vi "RT_Lissajou_fit_Oct.vi"() -> ()   [LabVIEW 2019]
uses:
  <vilib>/Platform/TimedLoop/XDataNode/timing_clust.ctl
  <vilib>/Platform/TimedLoop/XDataNode/nitl_modes.ctl
  <vilib>/Platform/TimedLoop/XDataNode/wakeup.ctl
  <vilib>/FPGAPlugInAG/myRIO-1900/niLvFpga_Open_myRIO-1900.vi
  <vilib>/rvi/interface/common/dynamic/niFpgaDynamicAddResources.vi
  <vilib>/Utility/error.llb/Error Cluster From Error Code.vi
  <vilib>/rvi/errors/niLvFpgaAdjustHostInterfaceError.vi
  <vilib>/gmath/NumericalOptimization/Nonlinear Curve Fit LM.vi
  <vilib>/platform/TimedLoop/XDataNode/XDataNode.xnode
  <vilib>/rvi/interface/nirviOpenFPGA/nirviOpenFPGA.xnode
  FPGA Bitfiles/studentchallenge_FPGATarget_FPGA1RADC1WDAC2A_GeAN6BgpSew.lvbitx
  <vilib>/rvi/interface/nirviReadWriteControl/nirviReadWriteControl.xnode
  <vilib>/Platform/TimedLoop/XDataNode/XDNodeRunTimeDep.lvlib
  <vilib>/gmath/NI_Gmath.lvlib
  <vilib>/Analysis/NI_AALBase.lvlib
  <vilib>/rvi/interface/Simulation/niFpgaSimulationCallBeginRW.vi
  NiFpgaLv.dll
panel:
  out "Fit":cluster{"X":dbl[], "Y":dbl[]}[](graph)
  out "Fit parameters":dbl[](array[numeric])=[0.5568165492992482, 1.080914000787513, 2.5775367916302736, 1.4146358342436716, -0.5221777499831268]
  out "?":dbl(graph)=3.104248046875
  out "Finished Late? [i-1]":bool
  out "?":dbl(graph)=1.22314453125
  in  "stop":bool
  out "Lissajou":cluster{"X":dbl[], "Y":dbl[]}[](graph)
  in  "Loop time (us)":i64=2000
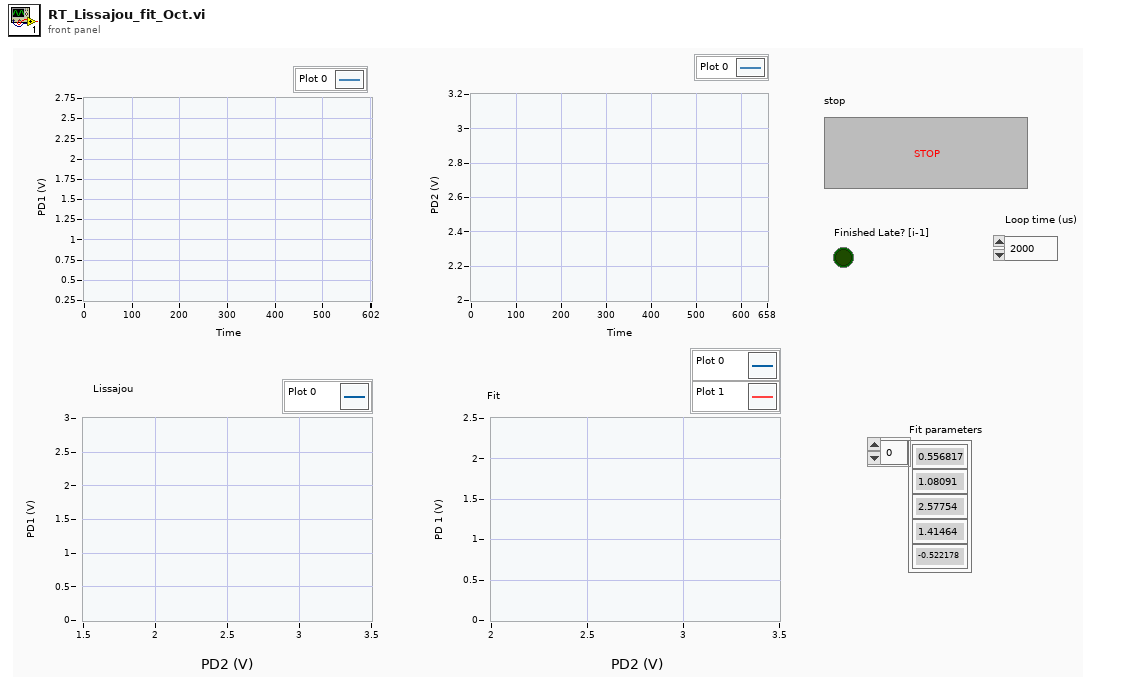
[diagram p1: front panel]
types:
  T1 = typedef "XDNodeRunTimeDep.lvlib/timing_clust.ctl" = cluster{"Expected End [f-1]":u64, "Actual End [f-1]":u64, "Finished Late? [f-1]":bool, "Expected End [i-1]":u64, "Actual End [i-1]":u64, "Finished Late? [i-1]":bool, "Expected Start [i]":u64, "Actual Start [i]":u64, "Expected Start [f]":u64, "Actual Start [f]":u64, "Source Name":string, "Structure Name":string, "Period":i64, "Deadline":i64, "Offset":i64, "Start":i64, "Priority":i32, "Timeout":i32, "Mode":T2, "Wakeup Reason":T3, "Error":errorcluster, "Source Type":string, "Secondary Source Type":string, "Global End Time":u64, "Global Start Time":u64, "Frame Duration":u64, "Iteration Duration":u64, "Assigned CPU":i32, "I/O Scan Engine Mode":u32}
  T2 = typedef "XDNodeRunTimeDep.lvlib/nitl_modes.ctl" = enum32{"No Change", "Process missed periods, maintain original phase", "Discard missed periods, maintain original phase", "Process missed periods, ignore original phase", "Discard missed periods, ignore original phase"}
  T3 = typedef "XDNodeRunTimeDep.lvlib/wakeup.ctl" = enum32{"Normal", "Aborted", "Asynchronous wakeup", "Timing source error", "Timed loop error", "Timeout"}
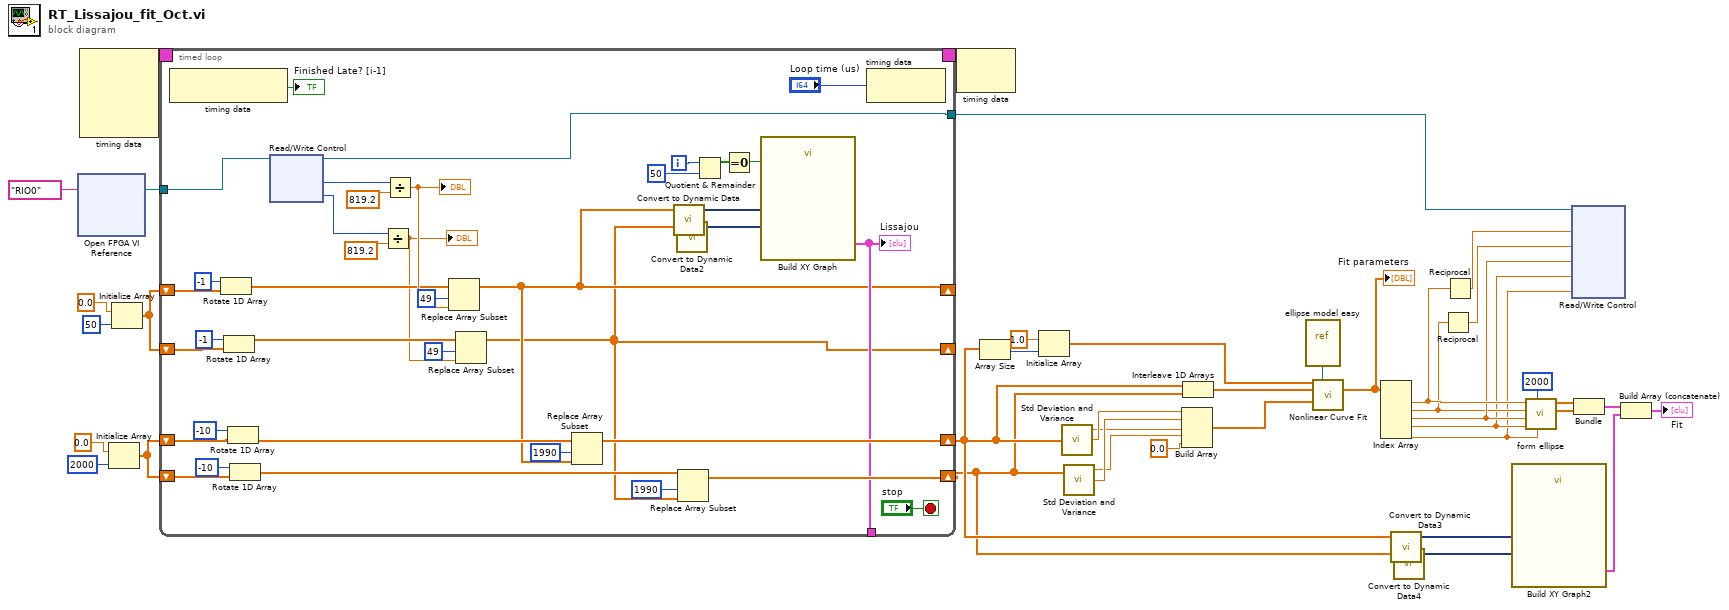
[diagram p0: block diagram]
diagram:
  n1 = xnode "Open FPGA VI Reference"("resource name"=tag "RIO0") -> ("FPGA VI Reference Out"=w37:refnum<k20>)  [unwired: 1 in, 1 out]
  n2 = node-c288() -> (w40:T1)  [unwired: 4 in]
  n3 = Initialize Array(0.0 ("element"), 2000 ("dimension size")) -> (w16:dbl[])
  n4 = Initialize Array(0.0 ("element"), 50 ("dimension size")) -> (w17:dbl[])
  n5 = timed-loop {
    timing: w40 -> [_]
    timing-out: [_] -> w39
    tunnel: w37 -> [w72]
    shift-right: [w43] -> _
    shift-left: w17 -> [w50]
    shift-right: [w44] -> _
    shift-left: w17 -> [w51]
    shift-right: [w49] -> w11
    shift-left: w16 -> [w48]
    shift-right: [w47] -> w12
    shift-left: w16 -> [w46]
    tunnel: [w45] -> _
    tunnel: [w41] -> w1
    i -> [w69]
    stop <- "stop" stop-if-true
    n6 = node-c288() -> (→"Finished Late? [i-1]":bool)  [unwired: 1 in]
    n7 = Rotate 1D Array(1:w51, 2:-1 ("n")) -> (0:w54:dbl[])
    n8 = Rotate 1D Array(1:w50, 2:-1 ("n")) -> (0:w53:dbl[])
    n9 = Rotate 1D Array(1:w46, 2:-10 ("n")) -> (0:w58:dbl[])
    n10 = Rotate 1D Array(1:w48, 2:-10 ("n")) -> (0:w59:dbl[])
    n11 = xnode "Read/Write Control"("FPGA VI Reference In"=w72) -> ("FPGA VI Reference Out"=w41:refnum<k20>, "PD1"=w77:u16, "PD2"=w74:u16)  [unwired: 1 in, 1 out]
    n12 = Divide(x=w74, y=819.2) -> (x/y=w52:dbl)
    "?" <- w52
    n13 = Divide(x=w77, y=819.2) -> (x/y=w55:dbl)
    "?" <- w55
    n14 = Replace Array Subset(array=w54, new element=w55, index=49) -> (w44:dbl[])
    n15 = Replace Array Subset(array=w53, new element=w52, index=49) -> (w43:dbl[])
    n16 = Replace Array Subset(array=w58, new element=w44, index=1990) -> (w47:dbl[])
    n17 = call "Convert to Dynamic Data"("Array"=w44) -> ("Dynamic Data Type"=w71:dynamicdata)  [unwired: 3 in]
    n18 = call "Convert to Dynamic Data2"("Array"=w43) -> ("Dynamic Data Type"=w70:dynamicdata)  [unwired: 3 in]
    n19 = Replace Array Subset(array=w59, new element=w43, index=1990) -> (w49:dbl[])
    n20 = Quotient & Remainder(x=w69, y=50) -> (x-y*floor(x/y)=w66:i32)  [unwired: 1 out]
    n21 = Equal To 0?(x=w66) -> (x = 0?=w67:bool)
    n22 = call "Build XY Graph"("Reset"=w67, "Y Input"=w70, "X Input"=w71) -> ("XY Graph"=w45:cluster{"X":dbl[], "Y":dbl[]}[])  [unwired: 7 in, 1 out]
    "Lissajou" <- w45
    n23 = node-c288("Loop time (us)") -> ()  [unwired: 1 out]
  }
  n24 = node-c288(w39) -> ()  [unwired: 1 out]
  n25 = Array Size(array=w12) -> (size(s)=w36:i32)
  n26 = Initialize Array(1.0 ("element"), w36) -> (w33:dbl[])
  n27 = call <vilib>:"Std Deviation and Variance.vi"("X"=w12) -> ("mean"=w23:dbl, "standard deviation"=w25:dbl)  [unwired: 1 in, 1 out]
  n28 = call <vilib>:"Std Deviation and Variance.vi"("X"=w11) -> ("mean"=w22:dbl, "standard deviation"=w24:dbl)  [unwired: 1 in, 1 out]
  n29 = Build Array(w25, w24, w23, w22, 0.0 ("element")) -> (w26:dbl[])
  n30 = Interleave 1D Arrays(w12, w11) -> (w32:dbl[])
  n31 = vi-ref "ellipse model easy.vi"() -> (w34:refnum<vi>)
  n32 = call-poly <vilib>:"Nonlinear Curve Fit.vi"("Y"=w33, "f(x,a)"=w34, "X"=w32, "initial parameters"=w26) -> ("best fit parameters"=w9:dbl[])  [unwired: 6 in, 5 out]
  "Fit parameters" <- w9
  n33 = Index Array(array=w9) -> (element #1=w7:dbl, element #2=w4:dbl, element #3=w5:dbl, element #4=w3:dbl, element #5=w2:dbl)  [unwired: 5 in]
  n34 = call "Convert to Dynamic Data3"("Array"=w12) -> ("Dynamic Data Type"=w14:dynamicdata)  [unwired: 3 in]
  n35 = call "Convert to Dynamic Data4"("Array"=w11) -> ("Dynamic Data Type"=w13:dynamicdata)  [unwired: 3 in]
  n36 = Reciprocal(x=w4) -> (1/x=w6:dbl)
  n37 = Reciprocal(x=w7) -> (1/x=w8:dbl)
  n38 = call "Build XY Graph2"("Y Input"=w13, "X Input"=w14) -> ("XY Graph"=w10:cluster{"X":dbl[], "Y":dbl[]}[])  [unwired: 8 in, 1 out]
  n39 = call "form ellipse.vi"("alpha"=w2, "samples"=2000, "y0"=w3, "x0"=w5, "b"=w4, "a"=w7) -> ("Y"=w28:dbl[], "X"=w29:dbl[])  [unwired: 4 in]
  n40 = xnode "Read/Write Control"("FPGA VI Reference In"=w1, "1/a"=w8, "1/b"=w6, "x0"=w5, "y0"=w3, "theta"=w2) -> ()  [unwired: 1 in, 2 out]
  n41 = Bundle("X"=w29, "Y"=w28) -> (w30:cluster{"X":dbl[], "Y":dbl[]})  [unwired: 1 in]
  n42 = Build Array (concatenate)(w30, w10) -> (→"Fit":cluster{"X":dbl[], "Y":dbl[]}[])
